vi "Write Loads.vi"(8 "error in (no error)":errorcluster, 10 "Loads":T1[](array[typedef]), 11 "ChromaAcLoad in":refnum<class "ChromaAcLoad.lvclass">) -> (0 "error out":errorcluster, 3 "ChromaAcLoad out":refnum<class "ChromaAcLoad.lvclass">)   [LabVIEW 2018, in "AcPwrPlugins.lvlib" / "ChromaAcLoad.lvclass"]
uses:
  ChromaAcLoad.lvclass
  TypeDefs/Load.ctl
  TypeDefs/LoadSettings.ctl
  TypeDefs/LC.ctl
  TypeDefs/LoadModes.ctl
  ChromaAcLoad.lvclass/ChromaAcLoad.ctl
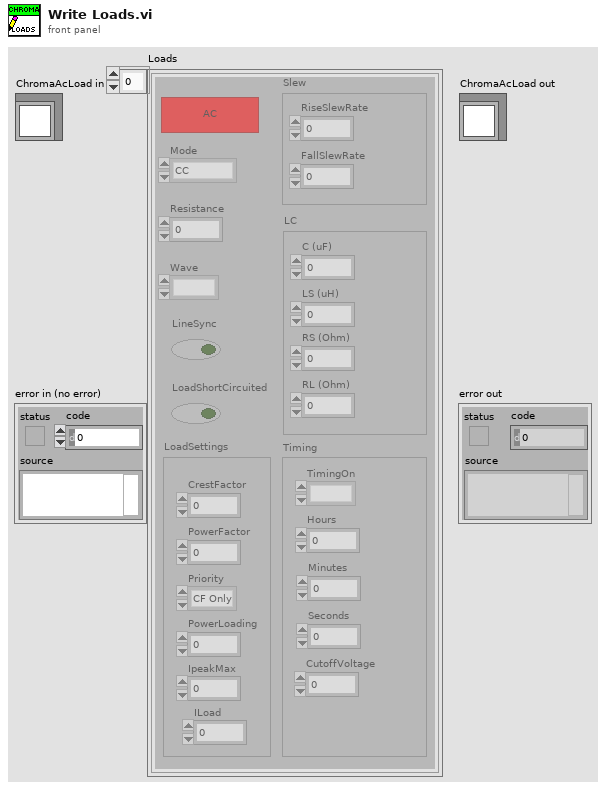
[diagram p1: front panel]
types:
  T1 = typedef "AcPwrPlugins.lvlib/ChromaAcLoad.lvclass/Load.ctl" = cluster{"AC/DC":bool, "Resistance":dbl, "LoadSettings":T2, "Wave":enum16{""}, "LineSync":bool, "LoadShortCircuited":bool, "LC":T3, "Timing":cluster{"TimingOn":enum16{""}, "Hours":u32, "Minutes":u32, "Seconds":dbl, "CutoffVoltage":dbl}, "Slew":cluster{"RiseSlewRate":i32, "FallSlewRate":i32}, "Mode":T4}
  T2 = typedef "AcPwrPlugins.lvlib/ChromaAcLoad.lvclass/LoadSettings.ctl" = cluster{"CrestFactor":dbl, "PowerFactor":dbl, "PowerLoading":dbl, "IpeakMax":dbl, "Priority":enum16{"CF Only", "PF Only", "Both (CF)", "Both (PF)"}, "ILoad":dbl}
  T3 = typedef "AcPwrPlugins.lvlib/ChromaAcLoad.lvclass/LC.ctl" = cluster{"C (uF)":i32, "LS (uH)":i32, "RL (Ohm)":dbl, "RS (Ohm)":dbl}
  T4 = typedef "AcPwrPlugins.lvlib/ChromaAcLoad.lvclass/LoadModes.ctl" = enum16{"CC", "CP", "CV", "CR", "RLC", "RLC CP", "Inrush", "Rectified"}
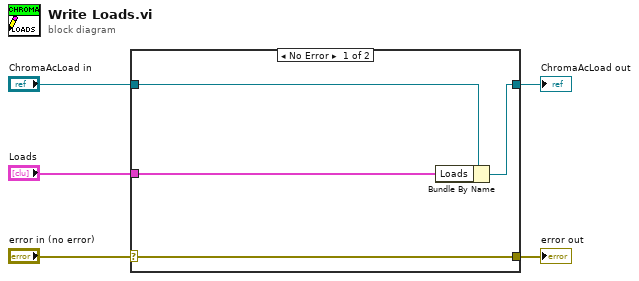
[diagram p0: block diagram]
diagram:
  n1 = case shown="No Error" "error in (no error)" {
    selector: "error in (no error)" -> [w9 w10]
    tunnel: [w9 w10] -> w4
    tunnel: [w7 w11] -> w2
    tunnel: "ChromaAcLoad in" -> [w8 w11]
    tunnel: "Loads" -> [w6 _]
    frame No Error {
      n2 = Bundle By Name(cluster=w8, "Loads"=w6) -> (w7:refnum<class "ChromaAcLoad.lvclass">)
    }
    frame Error {
    }
  }
  "error out" <- w4
  "ChromaAcLoad out" <- w2
